vi "DebugUtility_MemoryInspector.vi"() -> ()   [LabVIEW 2020]
uses:
  <resource>/objmgr/nisysapi.rc
panel:
  in  "Stop":bool
  out "Memory(%)":sgl(graph)
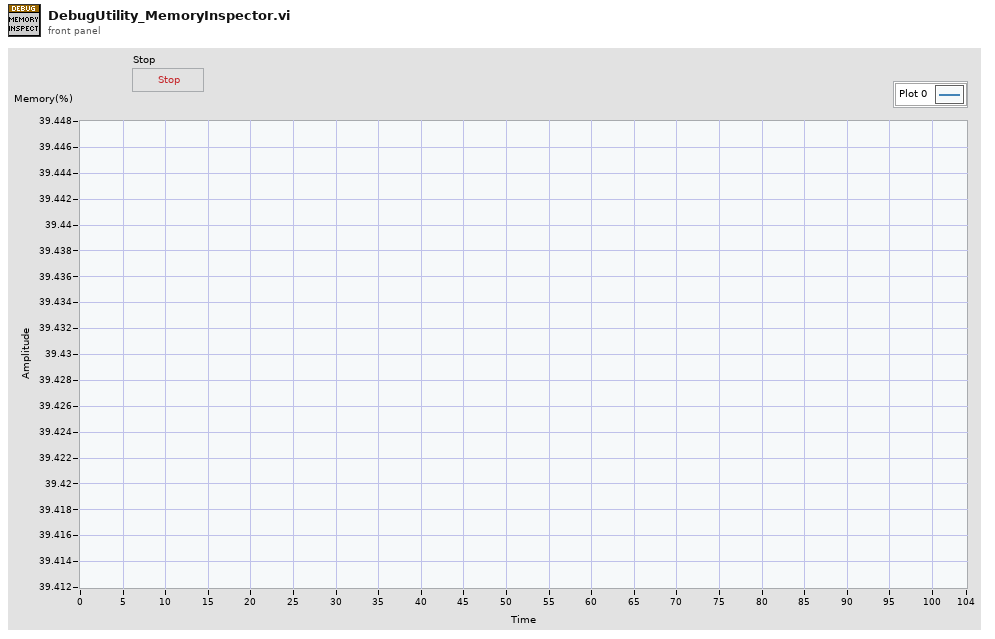
[diagram p1: front panel]
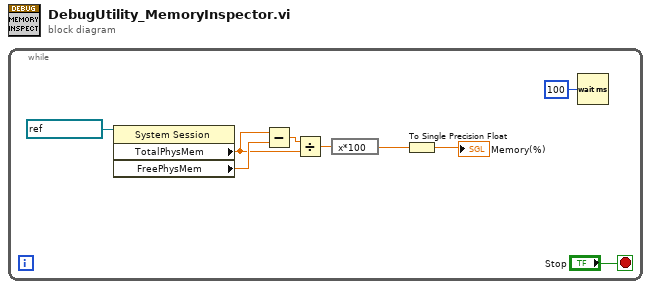
[diagram p0: block diagram]
diagram:
  n1 = while {
    stop <- "Stop" stop-if-true
    n2 = property class="System Session"(reference=refnum<k21> "localhost" ("System Session")) -> ("TotalPhysMem"=w7:dbl, "FreePhysMem"=w8:dbl)  [unwired: 1 in, 2 out]
    n3 = Subtract(x=w7, y=w8) -> (x-y=w9:dbl)
    n4 = Divide(x=w9, y=w7) -> (x/y=w6:dbl)
    n5 = expression code="x*100"(w6) -> (w4:dbl)
    n6 = To Single Precision Float(number=w4) -> (single precision float=→"Memory(%)":sgl)
    n7 = Wait (ms)(milliseconds to wait=u32 100) -> ()  [unwired: 1 out]
  }
